vi "Exit-all-clients.vi"(8 "error in (no error)":errorcluster, 11 "ModComm in":T1) -> (0 "error out":errorcluster, 3 "ModComm out":T1)   [LabVIEW 2013, in "SLMServer.lvlib" / "SLMServer.lvclass"]
uses:
  SLMServer.lvclass
  Object-reference.ctl
  SA-SLMAPI/Sources/Base-actions.ctl
  Supported-module-types.ctl
  SA-SLMAPI/Sources/Action/Action.lvclass
  SA-SLMAPI/SLMAPI.lvlib
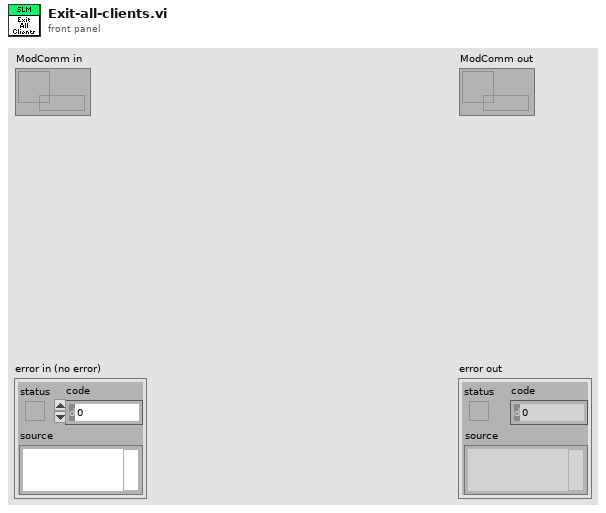
[diagram p1: front panel]
types:
  T1 = typedef "SLMServer.lvlib/SLMServer.lvclass/Object-reference.ctl" = refnum<data-value>
  T2 = typedef "SLMServer.lvlib/SLMServer.lvclass/Supported-module-types.ctl" = enum16{"SLMControl", "PowderDeposition", "CameraVision", "Server", "All", "StrategyParser", "MaterialCharacterization", "StatusMonitor", "SLMSimulation", "LaserCharacterization"}
  T3 = typedef "SLMAPI.lvlib/Base-actions.ctl" = enum16{"Idle", "Initialize", "Load settings", "Load file", "Activate", "Start", "Pause", "Stop", "Repeat", "Reset", "Exit"}
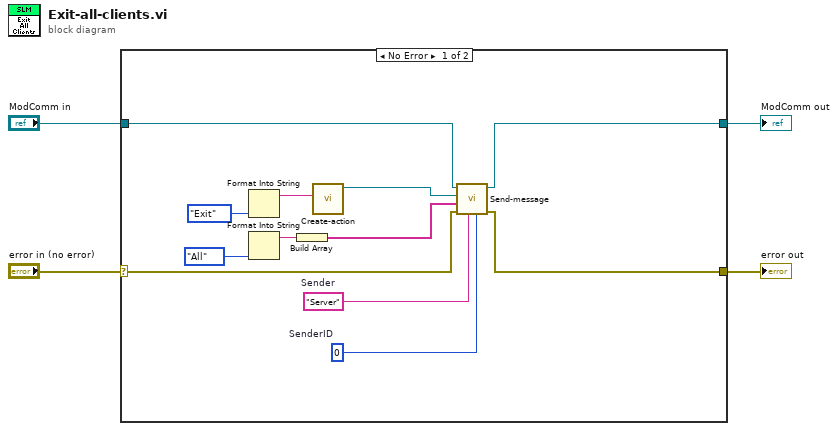
[diagram p0: block diagram]
diagram:
  n1 = case shown="No Error" "error in (no error)" {
    selector: "error in (no error)" -> [w8 w18]
    tunnel: [w7 w18] -> w3
    tunnel: [w14 w17] -> w1
    tunnel: "ModComm in" -> [w15 w17]
    frame No Error {
      w6 = 0  # SenderID
      w5 = "Server"  # Sender
      n2 = Format Into String(Base-actions."Exit" ("Action")) -> (resulting string=w16:string)  [unwired: 3 in, 1 out]
      n3 = Format Into String(Supported-module-types."All" ("Module type")) -> (resulting string=w10:string)  [unwired: 3 in, 1 out]
      n4 = Build Array(w10) -> (w9:string[])
      n5 = call "Create-action.vi"("Action"=w16) -> ("Action out"=w13:refnum<class "Action.lvclass">)  [unwired: 9 in, 1 out]
      n6 = call "Send-message.vi"("SenderID"=w6, "Sender"=w5, "error in (no error)"=w8, "Receivers"=w9, "Message"=w13, "Server in"=w15) -> ("error out"=w7:errorcluster, "Server out"=w14:T1)  [unwired: 4 in]
    }
    frame Error {
    }
  }
  "error out" <- w3
  "ModComm out" <- w1
